vi "Angulo_Horario (w).vi"(1 "Hora Solar":dbl) -> (0 "Ángulo Horario (w)":dbl(knob) scale=0.0..10.0)   [LabVIEW 2020]
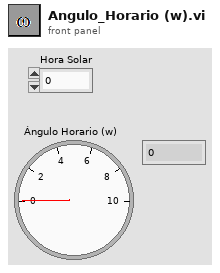
[diagram p1: front panel]
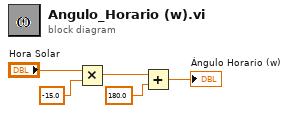
[diagram p0: block diagram]
diagram:
  n1 = Multiply(x="Hora Solar", y=-15.0) -> (x*y=w2:dbl)
  n2 = Add(x=w2, y=180.0) -> (x+y=→"Ángulo Horario (w)":dbl)
